vi "update config UI.vi"(8 "error in (no error)":errorcluster, 9 "config ui refs":T1, 10 "engine in":refnum<class "Engine Parent Editor Node.lvclass">, 11 "shared memory editor node in":refnum<class "module editor node.lvclass">) -> (0 "error out":errorcluster, 2 "engine out":refnum<class "Engine Parent Editor Node.lvclass">, 3 "shared memory editor node out":refnum<class "module editor node.lvclass">)   [LabVIEW 2013, in "Shared Memory editor node.lvclass"]
uses:
  Shared Memory editor node.lvclass
  <vilib>/NI/DCAF/Tag Editor Core/Configuration Editor/Classes/Module editor node/module editor node.lvclass
  ui controls config.ctl
  <vilib>/NI/DCAF/Tag Editor Core/Configuration Editor/Classes/Engine Parent/Engine Parent Editor Node.lvclass
  <vilib>/Utility/miscctls.llb/LVRowAndColumnTypeDef.ctl
  <vilib>/NI/DCAF/Tag Editor Core/Configuration Editor/Classes/Engine Parent/read engine configuration.vi
  <vilib>/NI/DCAF/Tag Editor Core/Configuration Editor/Classes/Engine Parent/write engine configuration.vi
  <vilib>/NI/Module Execution Interface/Engine Configuration/engine configuration.lvclass
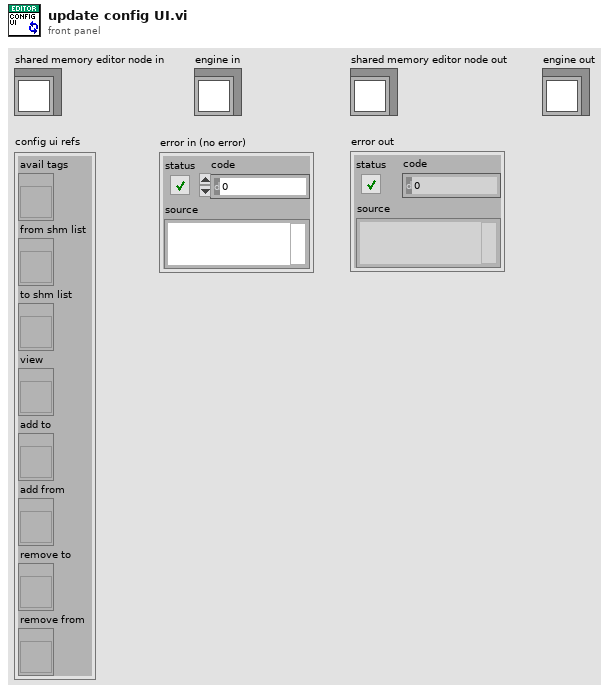
[diagram p1: front panel]
types:
  T1 = typedef "Shared Memory editor node.lvclass/ui controls config.ctl" = cluster{"avail tags":refnum<vi>, "from shm list":refnum<vi>, "to shm list":refnum<vi>, "view":refnum<vi>, "add to":refnum<vi>, "add from":refnum<vi>, "remove to":refnum<vi>, "remove from":refnum<vi>}
  T2 = typedef "LVRowAndColumnTypeDef.ctl" = cluster{"Row":i32, "Column":i32}
  T3 = enum8{"Enabled", "Disabled", "Disabled and Grayed Out"}
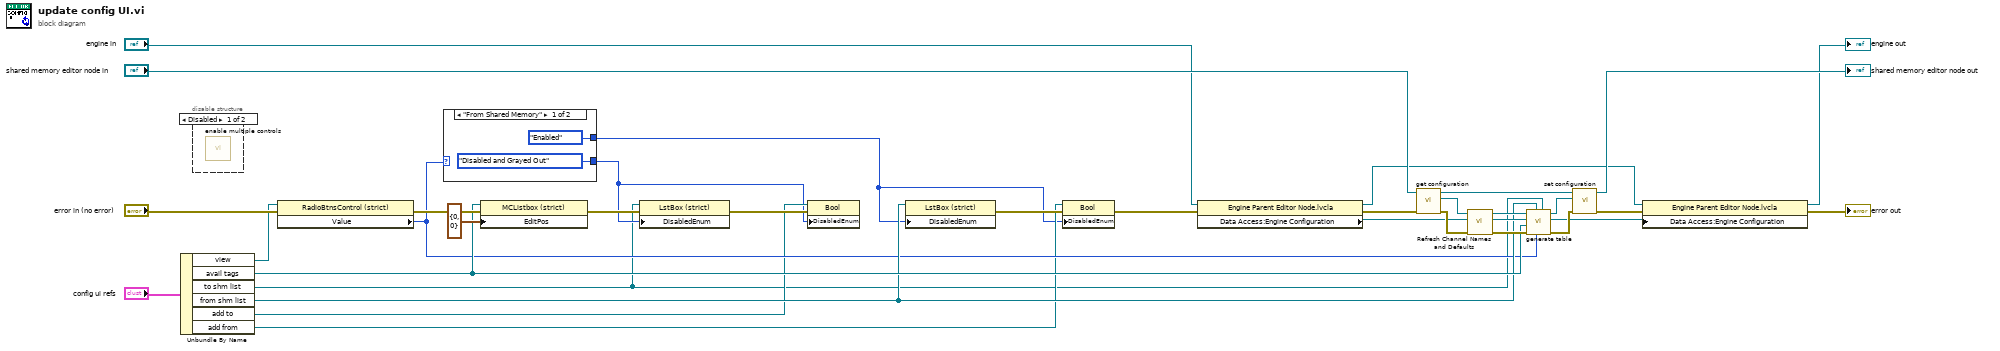
[diagram p0: block diagram]
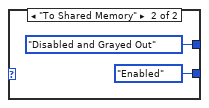
[diagram p3: hidden frame]
diagram:
  n1 = Unbundle By Name("config ui refs") -> ("view"=w31:refnum<vi>, "avail tags"=w16:refnum<vi>, "to shm list"=w1:refnum<vi>, "from shm list"=w15:refnum<vi>, "add to"=w7:refnum<vi>, "add from"=w4:refnum<vi>)
  n2 = disable-structure shown="Disabled" {
    frame Disabled {
      n3 = call "enable multiple controls.vi"() -> ()  [unwired: 9 in, 3 out]
    }
    frame Enabled {
    }
  }
  n4 = property class="RadioBtnsControl (strict)"(reference=w31, error in="error in (no error)") -> (error out=w30:errorcluster, "Value"=w9:enum32{"From Shared Memory", "To Shared Memory"})  [unwired: 1 out]
  n5 = case shown="\"From Shared Memory\"" w9 {
    tunnel: [T3."Enabled" ("Disabled") T3."Disabled and Grayed Out" ("Disabled")] -> w3
    tunnel: [T3."Disabled and Grayed Out" ("Disabled") T3."Enabled" ("Disabled")] -> w2
    frame "From Shared Memory" {
    }
    frame "To Shared Memory" {
    }
  }
  n6 = property on="Property Node" class="MCListbox (strict)"(reference=w16, error in=w30, "EditPos"=T2 {"Row"=0, "Column"=0} ("Edit Position")) -> (error out=w33:errorcluster)  [unwired: 1 out]
  n7 = property on="Property Node" class="LstBox (strict)"(reference=w1, error in=w33, "DisabledEnum"=w2) -> (error out=w8:errorcluster)  [unwired: 1 out]
  n8 = property on="Property Node" class="Bool"(reference=w7, error in=w8, "DisabledEnum"=w2) -> ()  [unwired: 2 out]
  n9 = property on="Property Node" class="LstBox (strict)"(reference=w15, "DisabledEnum"=w3) -> (error out=w6:errorcluster)  [unwired: 1 in, 1 out]
  n10 = property on="Property Node" class="Bool"(reference=w4, error in=w6, "DisabledEnum"=w3) -> (error out=w5:errorcluster)  [unwired: 1 out]
  n11 = property class="Engine Parent Editor Node.lvcla"(reference="engine in", error in=w5) -> (reference out=w12:refnum<class "Engine Parent Editor Node.lvclass">, error out=w22:errorcluster, "Data Access:Engine Configuration"=w21:refnum<class "engine configuration.lvclass">)
  n12 = call "get configuration.vi"("error in (no error)"=w22, "shared memory editor node in"="shared memory editor node in") -> ("error out"=w26:errorcluster, "shm configuration out"=w27:refnum<class "Shared Memory configuration.lvclass">, "shared memory editor node out"=w28:refnum<class "module editor node.lvclass">)  [unwired: 7 in]
  n13 = call "Refresh Channel Names and Defaults.vi"("error in (no error)"=w26, "engine configuration in"=w21, "SHM configuration in"=w27) -> ("error out"=w19:errorcluster, "engine configuration out"=w35:refnum<class "engine configuration.lvclass">, "SHM configuration out"=w20:refnum<class "Shared Memory configuration.lvclass">)  [unwired: 6 in]
  n14 = call "generate table.vi"("to cvt"=w1, "View"=w9, "from cvt"=w15, "error in"=w19, "avail tags"=w16, "engine configuration in"=w35, "shm config in"=w20) -> ("error out"=w17:errorcluster, "engine configuration out"=w13:refnum<class "engine configuration.lvclass">, "shm config out"=w18:refnum<class "Shared Memory configuration.lvclass">)  [unwired: 2 in]
  n15 = call "set configuration.vi"("error in (no error)"=w17, "shm configuration in"=w18, "shared memory editor node in"=w28) -> ("error out"=w14:errorcluster, "shared memory editor node out"=→"shared memory editor node out":refnum<class "module editor node.lvclass">)  [unwired: 7 in]
  n16 = property class="Engine Parent Editor Node.lvcla"(reference=w12, error in=w14, "Data Access:Engine Configuration"=w13) -> (reference out=→"engine out":refnum<class "Engine Parent Editor Node.lvclass">, error out=→"error out":errorcluster)
